vi "NetComm_CAN_OpenStreamSession.vi"(8 "error in (no error)":errorcluster, 9 "Max Messages":u32=512, 10 "Message ID Mask":u32=536870911 format="%.0x", 11 "Message ID":u32 format="%.0x") -> (0 "error out":errorcluster, 3 "Session Handle":u32)   [LabVIEW 2017]
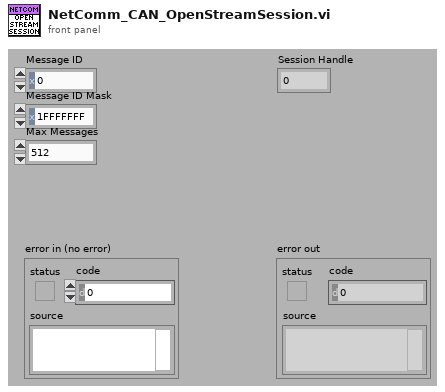
[diagram p1: front panel]
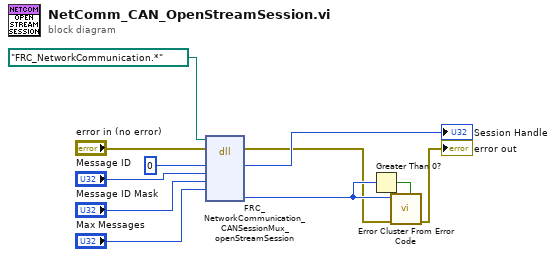
[diagram p0: block diagram]
diagram:
  n1 = dll-call lib="FRC_NetworkCommunication.*" fn="FRC_NetworkCommunication_CANSessionMux_openStreamSession"(path in=path "FRC_NetworkCommunication.*", error in="error in (no error)", "sessionHandle"=u32 0, "messageID"="Message ID", "messageIDMask"="Message ID Mask", "maxMessages"="Max Messages") -> (error out=w2:errorcluster, "sessionHandle"=→"Session Handle":u32, "status"=w8:i32)  [unwired: 6 in, 1 out]
  n2 = Greater Than 0?(x=w8) -> (x > 0?=w9:bool)
  n3 = call <vilib>:"Error Cluster From Error Code.vi"("is warning? (False)"=w9, "error in (no error)"=w2, "error code (0)"=w8) -> ("error out"=→"error out":errorcluster)  [unwired: 1 in, 5 out]
